vi "XY Go.vi"(8 "error in (no error)":errorcluster, 9 "Speed":dbl, 10 "XY":dbl[](array[numeric]), 11 "Gantry 2":refnum<k24>) -> (0 "error out":errorcluster, 3 "Gantry 3":refnum<k24>)   [LabVIEW 2020, in "A3200.lvclass"]
uses:
  A3200.lvclass
  C:/Program Files (x86)/Aerotech/A3200/LabVIEW/2010/Bin/Aerotech.A3200.dll
  Program Files (x86)/Aerotech/A3200/LabVIEW/2010/Bin/Aerotech.A3200.dll
  Aerotech.lvlib
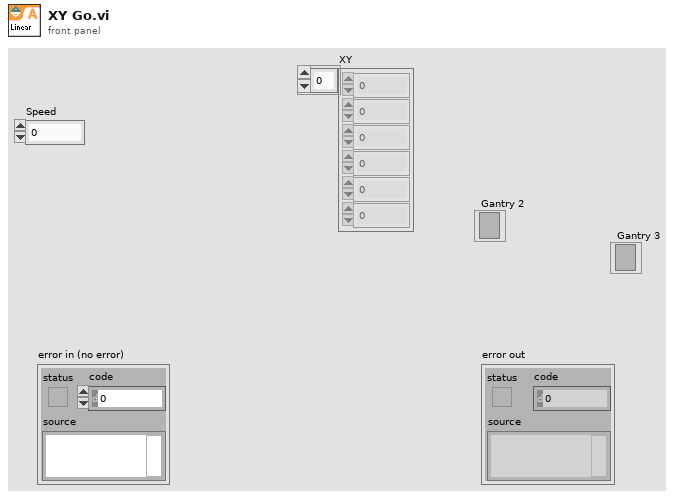
[diagram p1: front panel]
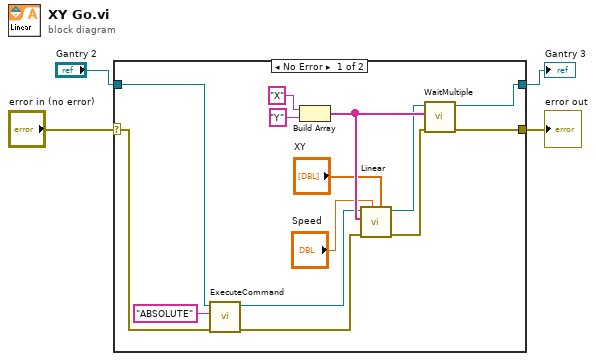
[diagram p0: block diagram]
diagram:
  n1 = case shown="No Error" "error in (no error)" {
    selector: "error in (no error)" -> [w6 w20]
    tunnel: [w16 w20] -> w3
    tunnel: [w15 w19] -> w1
    tunnel: "Gantry 2" -> [w9 w19]
    frame No Error {
      n2 = call "ExecuteCommand.vi"("error in (no error)"=w6, "Command Code"="ABSOLUTE", "controller in"=w9) -> ("error out"=w5:errorcluster, "controller out"=w8:refnum<k24>)  [unwired: 6 in, 1 out]
      n3 = Build Array("X" ("format string"), "Y" ("format string")) -> (w14:string[])
      n4 = call "Linear.vi"("distances"="XY", "speed"="Speed", "error in (no error)"=w5, "axis names"=w14, "controller in"=w8) -> ("error out"=w13:errorcluster, "controller out"=w10:refnum<k24>)  [unwired: 5 in]
      n5 = call "WaitMultiple.vi"("error in (no error)"=w13, "axis names"=w14, "controller in"=w10) -> ("error out"=w16:errorcluster, "controller out"=w15:refnum<k24>)  [unwired: 6 in, 1 out]
    }
    frame Error {
    }
  }
  "error out" <- w3
  "Gantry 3" <- w1
